vi "LoggingOperation.vi"(8 "Operation":T2, 10 "Data":variant, 11 "Name":T1) -> (3 "Log String":string)   [LabVIEW 2017]
uses:
  LogOperation.ctl
  DataNames.ctl
  <vilib>/Utility/Data Type/NI_Data Type.lvlib
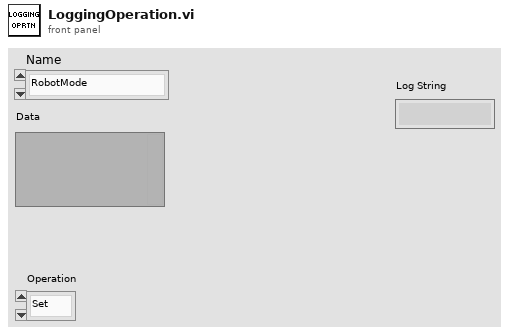
[diagram p1: front panel]
types:
  T1 = typedef "DataNames.ctl" = enum16{"RobotMode", "FMSConnected", "DriveLeft", "DriveRight", "EncoderLeft", "EncoderRight", "Angle", "LocationX", "LocationY", "CPU", "DriveOperation", "Battery"}
  T2 = typedef "LogOperation.ctl" = enum16{"Set", "Get All", "Get Headers"}
  T3 = typedef "NI_Data Type.lvlib/Data Type.ctl" = enum8{"Invalid Type", "Void", "I8", "I16", "I32", "I64", "U8", "U16", "U32", "U64", "Single Float", "Double Float", "Extended Float", "Single Complex", "Double Complex", "Extended Complex", "Enum U8", "Enum U16", "Enum U32", "Enum U64", "Single Float With Unit", "Double Float With Unit", "Extended Float With Unit", "Single Complex with Unit", "Double Complex with Unit", "Extended Complex with Unit", "Boolean", "String", "Path", "Picture", "Tag", "Array", "Cluster", "Variant", "LV Variant", "Waveform", "Timestamp", "Digital Waveform", "Digital Data", "ExpressData", "Refnum", "External Data", "VI", "Poly VI", "LabVIEW Class Instance", "Fixed Point"}
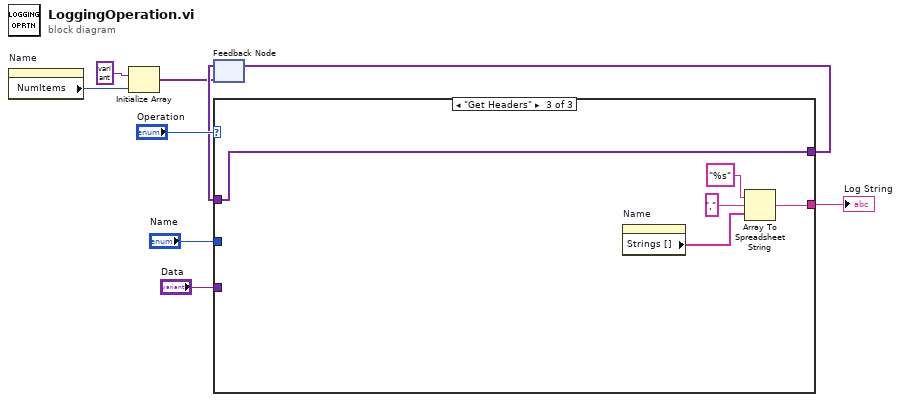
[diagram p0: block diagram]
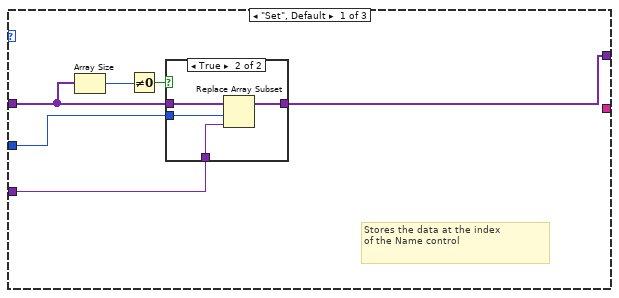
[diagram p2: hidden frame]
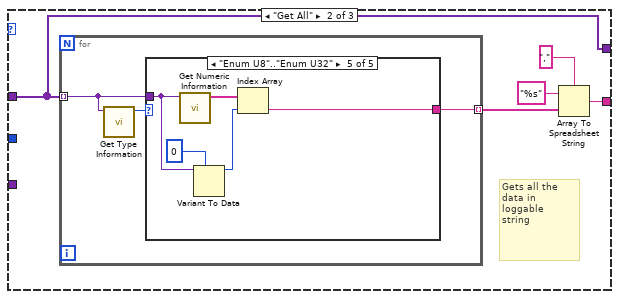
[diagram p4: hidden frame]
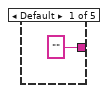
[diagram p5: hidden frame]
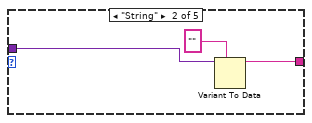
[diagram p6: hidden frame]
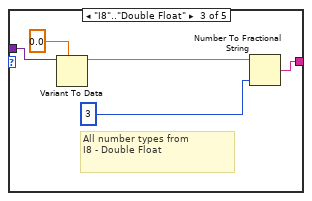
[diagram p7: hidden frame]
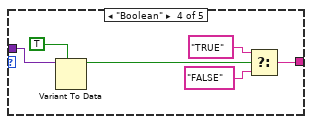
[diagram p8: hidden frame]
diagram:
  n1 = property on="Name" class="Enum (strict)"() -> ("NumItems"=w3:u32)  [unwired: 2 in, 2 out]
  n2 = Initialize Array(variant, w3) -> (w1:variant[])
  n3 = feedback #1(w1) -> (w8:variant[])
  n4 = case shown="\"Get Headers\"" "Operation" {
    tunnel: w8 -> [w13 w22 w49]
    tunnel: [w14 w22 w49] -> w7
    tunnel: "Data" -> [w15 _ _]
    tunnel: [_ w24 w51] -> w5
    tunnel: "Name" -> [w12 _ _]
    frame "Set", Default {
      # "Stores the data at the index\nof the Name control"
      n5 = Array Size(array=w13) -> (size(s)=w11:i32)
      n6 = Not Equal To 0?(x=w11) -> (x != 0?=w10:bool)
      n7 = case shown="True" w10 {
        tunnel: w15 -> [_ w20]
        tunnel: w12 -> [_ w19]
        tunnel: [w16 w18] -> w14
        tunnel: w13 -> [w16 w17]
        frame False {
        }
        frame True {
          n8 = Replace Array Subset(array=w17, new element=w20, index=w19) -> (w18:variant[])
        }
      }
    }
    frame "Get All" {
      # "Gets all the\ndata in\nloggable\nstring"
      n9 = for {
        tunnel: w22 -> [w27] mode=indexing
        tunnel: [w28] -> w23 mode=indexing
        n10 = call <vilib>:"Get Type Information.vi"("Variant"=w27) -> ("Type"=w26:T3)  [unwired: 6 in, 4 out]
        n11 = case shown="\"Enum U8\"..\"Enum U32\"" w26 {
          tunnel: ["" ("Name") w32 w34 w39 w45] -> w28
          tunnel: w27 -> [_ w30 w33 w38 w44]
          frame Default {
          }
          frame "String" {
            n12 = Variant To Data(type="" ("Name"), Variant=w30) -> (data=w32:string)  [unwired: 1 in, 1 out]
          }
          frame "I8".."Double Float" {
            # "All number types from\nI8 - Double Float"
            n13 = Variant To Data(type=0.0, Variant=w33) -> (data=w36:dbl)  [unwired: 1 in, 1 out]
            n14 = Number To Fractional String(number=w36, precision (6)=i16 3) -> (F-format string=w34:string)  [unwired: 2 in]
          }
          frame "Boolean" {
            n15 = Variant To Data(type=TRUE, Variant=w38) -> (data=w42:bool)  [unwired: 1 in, 1 out]
            n16 = Select(t="TRUE" ("format string"), s=w42, f="FALSE" ("format string")) -> (s? t:f=w39:string)
          }
          frame "Enum U8".."Enum U32" {
            n17 = call <vilib>:"Get Numeric Information.vi"("Variant"=w44) -> ("Enum Names"=w48:string[])  [unwired: 7 in, 3 out]
            n18 = Variant To Data(type=u32 0 ("milliseconds to wait"), Variant=w44) -> (data=w46:u32)  [unwired: 1 in, 1 out]
            n19 = Index Array(array=w48, index=w46) -> (element=w45:string)
          }
        }
      }
      n20 = Array To Spreadsheet String(delimiter (Tab)=",", array=w23, 3:"%s" ("format string")) -> (spreadsheet string=w24:string)
    }
    frame "Get Headers" {
      n21 = property on="Name" class="Enum (strict)"() -> ("Strings []"=w50:string[])  [unwired: 2 in, 2 out]
      n22 = Array To Spreadsheet String(delimiter (Tab)=",", array=w50, 3:"%s" ("format string")) -> (spreadsheet string=w51:string)
    }
  }
  "Log String" <- w5
  n23 = feedback-in #1(w7) -> ()
